vi "PXI_Host_I16_Write_OldMethod_Benchmark.vi"() -> ()   [LabVIEW 2018]
uses:
  <vilib>/Platform/TimedLoop/XDataNode/timing_clust.ctl
  <vilib>/Platform/TimedLoop/XDataNode/nitl_modes.ctl
  <vilib>/Platform/TimedLoop/XDataNode/wakeup.ctl
  <vilib>/NI/LVFPGA Adv Session Resources/OpenByNameSubVI.vi
  <vilib>/rvi/interface/common/dynamic/niFpgaEscapeDelimiterAndNull.vi
  <vilib>/Utility/error.llb/Error Cluster From Error Code.vi
  <vilib>/rvi/errors/niLvFpgaAdjustHostInterfaceError.vi
  <vilib>/FPGAPlugInAG/Dynamic/niLvFpga_Close_Dynamic.vi
  <vilib>/platform/TimedLoop/XDataNode/XDataNode.xnode
  <vilib>/NI/LVFPGA Adv Session Resources/OpenByName.xnode
  <vilib>/rvi/interface/nirviReadWriteControl/nirviReadWriteControl.xnode
  <vilib>/rvi/interface/nirviCloseFPGA/nirviCloseFPGA.xnode
  NiFpgaLv.dll
  <vilib>/rvi/interface/Simulation/niFpgaSimulationCallBeginRW.vi
  <vilib>/NI/LVFPGA Adv Session Resources/LVFPGAAdvSessionResources.lvlib
  cRIO RT/FPGA Bitfile Register Operations/Scalar IO Operations/FPGA Register IO.lvlib
  <vilib>/Platform/TimedLoop/XDataNode/XDNodeRunTimeDep.lvlib
panel:
  out "Maximum(s)":dbl
  out "Standard deviation":dbl
  out "Waveform Graph":dbl[](graph)
  out "error out":errorcluster
  out "Execution time (s)":dbl
  # "Recorded time"
  # "3.37551E-5"
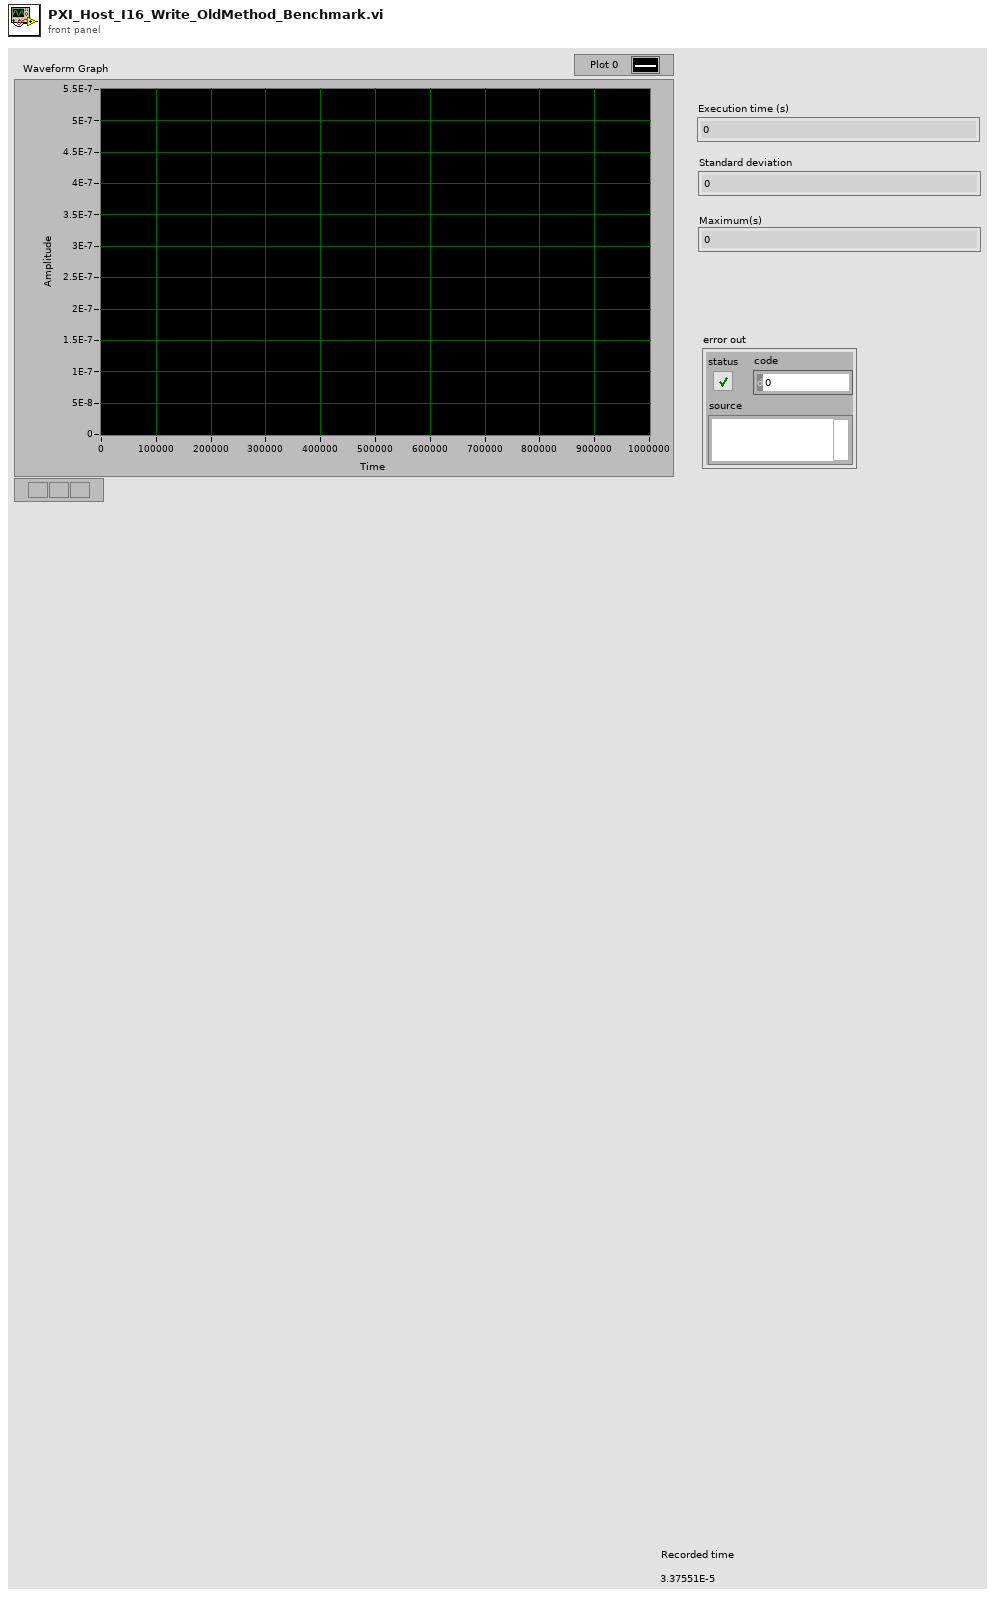
[diagram p1: front panel]
types:
  T1 = typedef "XDNodeRunTimeDep.lvlib/timing_clust.ctl" = cluster{"Expected End [f-1]":u64, "Actual End [f-1]":u64, "Finished Late? [f-1]":bool, "Expected End [i-1]":u64, "Actual End [i-1]":u64, "Finished Late? [i-1]":bool, "Expected Start [i]":u64, "Actual Start [i]":u64, "Expected Start [f]":u64, "Actual Start [f]":u64, "Source Name":string, "Structure Name":string, "Period":i64, "Deadline":i64, "Offset":i64, "Start":i64, "Priority":i32, "Timeout":i32, "Mode":T2, "Wakeup Reason":T3, "Error":errorcluster, "Source Type":string, "Secondary Source Type":string, "Global End Time":u64, "Global Start Time":u64, "Frame Duration":u64, "Iteration Duration":u64, "Assigned CPU":i32, "I/O Scan Engine Mode":u32}
  T2 = typedef "XDNodeRunTimeDep.lvlib/nitl_modes.ctl" = enum32{"No Change", "Process missed periods, maintain original phase", "Discard missed periods, maintain original phase", "Process missed periods, ignore original phase", "Discard missed periods, ignore original phase"}
  T3 = typedef "XDNodeRunTimeDep.lvlib/wakeup.ctl" = enum32{"Normal", "Aborted", "Asynchronous wakeup", "Timing source error", "Timed loop error", "Timeout"}
  T4 = cluster{"Name":string, "Depth":u32, "Write? (Deprecated:Use Implementation)":bool, "Physical Channel":u32, "Base Address":u32, "Data Width":u32, "Data Type":enum32{"Boolean", "I8", "I16", "I32", "I64", "U8", "U16", "U32", "U64", "FXP", "CustomControl", "SGL"}, "FXP Properties":variant, "Write Window Address":u32, "Implementation":enum16{"niFpgaTargetToHost", "niFpgaHostToTarget", "niFpgaPeerToPeerWriter", "niFpgaPeerToPeerReader", "niCoreTargetToHost", "niCoreHostToTarget"}, "Control Set":u32}[]
  T5 = cluster{"Name":string, "type":variant, "indicator?":bool}[]
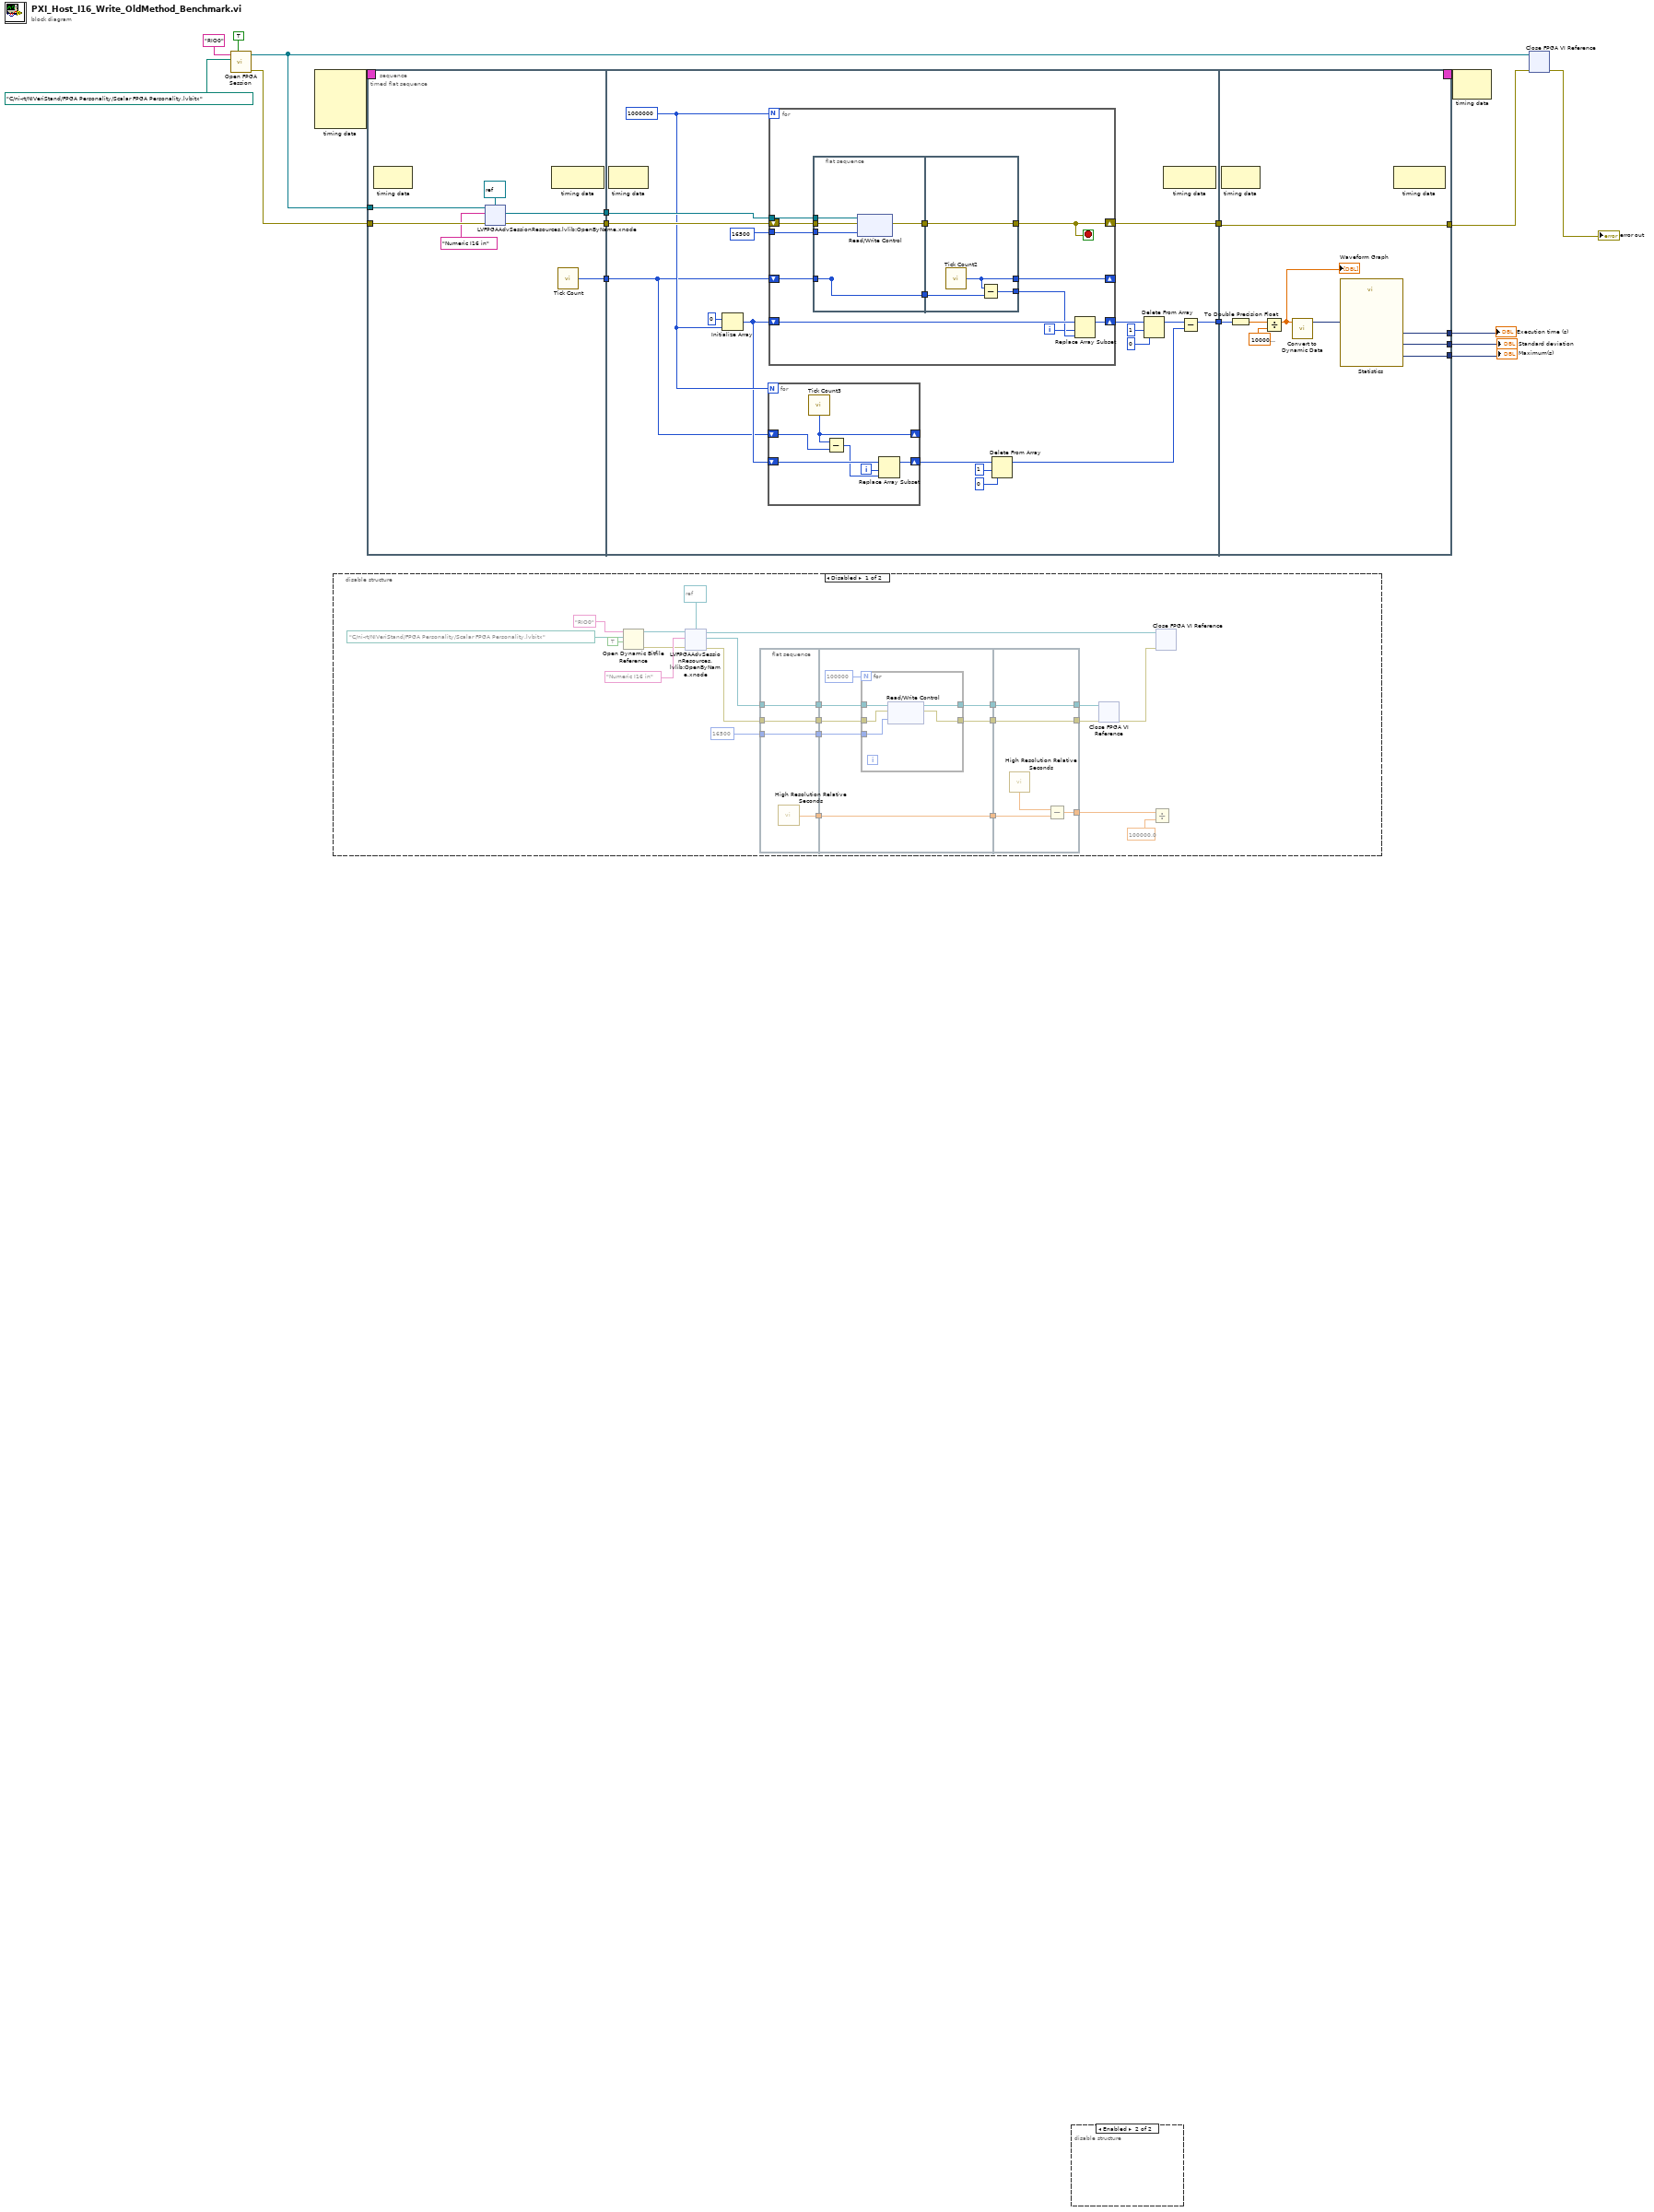
[diagram p0: block diagram]
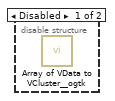
[diagram p3: hidden frame]
diagram:
  n1 = call "Open FPGA Session.vi"("run when loaded (T)"=TRUE, "bitfile path"=path "C:/ni-rt/NIVeriStand/FPGA Personality/Scalar FPGA Personality.lvbitx", "device address"="RIO0") -> ("error out"=w7:errorcluster, "bitfile reference out"=w1:refnum<k20>)  [unwired: 6 in, 1 out]
  n2 = node-c288() -> (w12:T1)  [unwired: 4 in]
  n3 = disable-structure shown="Disabled" {
    frame Disabled {
      n4 = Open Dynamic Bitfile Reference(0:"RIO0" ("Device address"), 1:path "C:/ni-rt/NIVeriStand/FPGA Personality/Scalar FPGA Personality.lvbitx" ("Bitfile path"), 2:TRUE ("Run When Loaded")) -> (5:w22:refnum<k20>, 8:w20:errorcluster)  [unwired: 2 in]
      n5 = xnode "LVFPGAAdvSessionResources.lvlib:OpenByName.xnode"("FPGA VI Reference in"=w22, "Resource name in"="Numeric I16 in", "Single resource reference type in"=refnum<k20> refnum ("Type"), "Error in"=w20) -> ("Single resource reference out"=w18:refnum<k20>, "Error out"=w19:errorcluster, "FPGA VI Reference out"=w14:refnum<k20>)
      n6 = flat-sequence {
        tunnel: [w39] -> w35
        tunnel: w18 -> [w38]
        tunnel: [w38] -> w34
        tunnel: [w37] -> w33
        tunnel: w19 -> [w37]
        tunnel: [w36] -> w32
        tunnel: i16 16500 ("Value") -> [w36]
        tunnel: [w45] -> w31
        tunnel: w35 -> [w45]
        tunnel: w34 -> [w44]
        tunnel: w33 -> [w43]
        tunnel: [w42] -> w30
        tunnel: [w41] -> w29
        tunnel: w32 -> [w40]
        tunnel: w31 -> [w55]
        tunnel: [w54] -> w28
        tunnel: w30 -> [w53]
        tunnel: [w53] -> w23
        tunnel: w29 -> [w52]
        tunnel: [w52] -> w16
        frame #0 {
          n7 = call <vilib>:"High Resolution Relative Seconds.vi"() -> ("relative seconds"=w39:dbl)
        }
        frame #1 {
          n8 = for {
            N: 100000 -> [_]
            tunnel: w44 -> [w51]
            tunnel: w43 -> [w50]
            tunnel: [w49] -> w42
            tunnel: [w48] -> w41
            tunnel: w40 -> [w47]
            n9 = xnode "Read/Write Control"("FPGA VI Reference In"=w51, "error in"=w50, "Value"=w47) -> ("FPGA VI Reference Out"=w48:refnum<k20>, "error out"=w49:errorcluster)
          }
        }
        frame #2 {
          n10 = call <vilib>:"High Resolution Relative Seconds.vi"() -> ("relative seconds"=w56:dbl)
          n11 = Subtract(x=w56, y=w55) -> (x-y=w54:dbl)
        }
      }
      n12 = xnode "Close FPGA VI Reference"("FPGA VI Reference In"=w16, "error in"=w23) -> ("error out"=w15:errorcluster)
      n13 = Divide(x=w28, y=100000.0) -> ()  [unwired: 1 out]
      n14 = xnode "Close FPGA VI Reference"("FPGA VI Reference In"=w14, "error in"=w15) -> ()  [unwired: 1 out]
    }
    frame Enabled {
    }
  }
  n15 = timed-sequence {
    timing: w12 -> [_]
    timing-out: [_] -> w11
    tunnel: w7 -> [w71]
    tunnel: [w77] -> w6
    tunnel: [w74] -> w4
    tunnel: [w73] -> w3
    tunnel: [w72] -> w2
    tunnel: w1 -> [w70]
    n16 = timed-flat-sequence {
      tunnel: [w84] -> w80
      tunnel: [w85] -> w79
      tunnel: [w87] -> w76
      tunnel: w71 -> [w83]
      tunnel: w70 -> [w86]
      tunnel: w80 -> [w119]
      tunnel: [w118] -> w78
      tunnel: w79 -> [w117]
      tunnel: w76 -> [w107]
      tunnel: [w104] -> w75
      tunnel: w78 -> [w157]
      tunnel: [w157] -> w77
      tunnel: w75 -> [w156]
      tunnel: [w154] -> w74
      tunnel: [w151] -> w73
      tunnel: [w150] -> w72
      frame #0 {
        n17 = node-c288() -> ()  [unwired: 1 in, 1 out]
        n18 = xnode "LVFPGAAdvSessionResources.lvlib:OpenByName.xnode"("FPGA VI Reference in"=w86, "Resource name in"="Numeric I16 in", "Single resource reference type in"=refnum<k20> refnum ("Type"), "Error in"=w83) -> ("Single resource reference out"=w85:refnum<k20>, "Error out"=w84:errorcluster)  [unwired: 1 out]
        n19 = node-c288() -> ()  [unwired: 1 in, 1 out]
        n20 = call "Tick Count"() -> ("Tick Count(Ticks)"=w87:u32)
      }
      frame #1 {
        w109 = 1000000
        n21 = node-c288() -> ()  [unwired: 1 in, 1 out]
        n22 = Initialize Array(u32 0, w109) -> (w108:u32[])
        n23 = for {
          N: w109 -> [_]
          shift-right: [w120] -> w110
          shift-left: w108 -> [w123]
          shift-right: [w125] -> _
          shift-left: w107 -> [w124]
          i -> [w121]
          n24 = call "Tick Count3"() -> ("Tick Count(Ticks)"=w125:u32)
          n25 = Subtract(x=w125, y=w124) -> (x-y=w122:u32)
          n26 = Replace Array Subset(array=w123, new element=w122, index=w121) -> (w120:u32[])
        }
        n27 = for {
          N: w109 -> [_]
          tunnel: w117 -> [w138]
          shift-right: [w136] -> _
          shift-left: w107 -> [w135]
          shift-right: [w131] -> w115
          shift-left: w108 -> [w133]
          shift-right: [w129] -> w118
          shift-left: w119 -> [w139]
          tunnel: i16 16500 ("Value") -> [w128]
          i -> [w130]
          stop <- w129 stop-if-true
          n28 = flat-sequence {
            tunnel: w139 -> [w143]
            tunnel: w138 -> [w141]
            tunnel: [w142] -> w137
            tunnel: [w144] -> _
            tunnel: w135 -> [w144]
            tunnel: [w144] -> w134
            tunnel: w128 -> [w140]
            tunnel: [w148] -> w129
            tunnel: w137 -> [w148]
            tunnel: [w147] -> w136
            tunnel: w134 -> [w146]
            tunnel: [w145] -> w132
            frame #0 {
              n29 = xnode "Read/Write Control"("FPGA VI Reference In"=w141, "error in"=w143, "Value"=w140) -> ("error out"=w142:errorcluster)  [unwired: 1 out]
            }
            frame #1 {
              n30 = call "Tick Count2"() -> ("Tick Count(Ticks)"=w147:u32)
              n31 = Subtract(x=w147, y=w146) -> (x-y=w145:u32)
            }
          }
          n32 = Replace Array Subset(array=w133, new element=w132, index=w130) -> (w131:u32[])
        }
        n33 = Delete From Array(array=w110, length=1, index=0) -> (array with subset deleted=w105:u32[])  [unwired: 1 out]
        n34 = Delete From Array(array=w115, length=1, index=0) -> (array with subset deleted=w106:u32[])  [unwired: 1 out]
        n35 = node-c288() -> ()  [unwired: 1 in, 1 out]
        n36 = Subtract(x=w106, y=w105) -> (x-y=w104:u32[])
      }
      frame #2 {
        n37 = node-c288() -> ()  [unwired: 1 in, 1 out]
        n38 = To Double Precision Float(number=w156) -> (double precision float=w153:dbl[])
        n39 = Divide(x=w153, y=1000000000.0) -> (x/y=w149:dbl[])
        "Waveform Graph" <- w149
        n40 = call "Convert to Dynamic Data"("Array"=w149) -> ("Dynamic Data Type"=w155:dynamicdata)  [unwired: 3 in]
        n41 = call "Statistics"("Signals"=w155) -> ("Standard Dev"=w151:dynamicdata, "Arithmetic Mean"=w154:dynamicdata, "Maximum"=w150:dynamicdata)  [unwired: 23 in, 1 out]
        n42 = node-c288() -> ()  [unwired: 1 in, 1 out]
      }
    }
  }
  "Execution time (s)" <- w4
  "Standard deviation" <- w3
  "Maximum(s)" <- w2
  n43 = disable-structure shown="Enabled" {
    frame Disabled {
      n44 = call <userlib>:"Array of VData to VCluster__ogtk.vi"() -> ()  [unwired: 10 in, 2 out]
    }
    frame Enabled {
    }
  }
  n45 = node-c288(w11) -> ()  [unwired: 1 out]
  n46 = xnode "Close FPGA VI Reference"("FPGA VI Reference In"=w1, "error in"=w6) -> ("error out"=→"error out":errorcluster)
